vi "View Song Library Request by Album.vi"(8 "error in (no error)":errorcluster, 9 "Artist":string, 10 "Album":string, 11 "MusicManagerActor in":refnum<class "MusicManagerActor.lvclass">) -> (0 "error out":errorcluster, 3 "MusicManagerActor out":refnum<class "MusicManagerActor.lvclass">)   [LabVIEW 2015, in "MusicManagerActor.lvlib" / "MusicManagerActor.lvclass"]
uses:
  MusicManagerActor.lvclass
  MusicManagerActor.lvclass/MusicManagerActor.ctl
  file/MusicElement/Album/Album.lvclass/Album.ctl
  file/MusicElement/MusicElementLibrary/SongLibrary/SongLibrary.lvclass
  SongBrowserActor/SongBrowserActor Messages/Display Song Library Msg/Display Song Library Msg.lvclass
  file/MusicElement/MusicElementLibrary/MusicLibrary/MusicLibrary.lvclass
  SongQueueActor/SongQueueActor Messages/Set Visibility Of Queue List Msg/Set Visibility Of Queue List Msg.lvclass
  file/MusicElement/Album/Album.lvclass
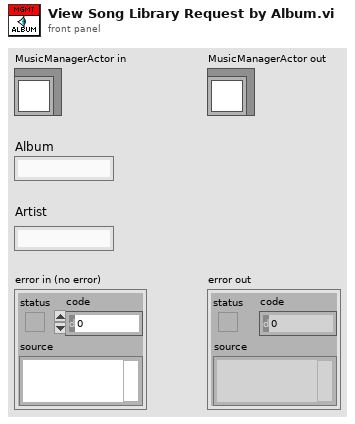
[diagram p1: front panel]
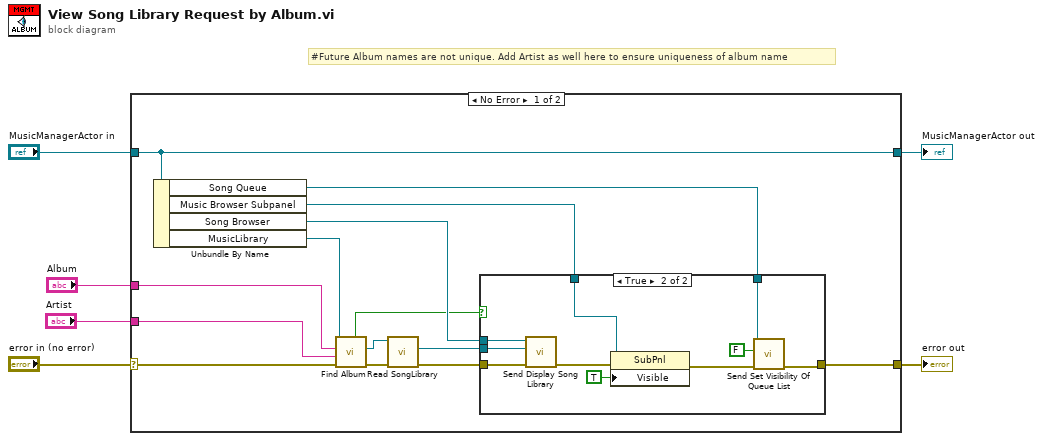
[diagram p0: block diagram]
diagram:
  # "#Future Album names are not unique. Add Artist as well here to ensure uniqueness of album name"
  n1 = case shown="No Error" "error in (no error)" {
    selector: "error in (no error)" -> [w16 w33]
    tunnel: [w19 w33] -> w5
    tunnel: [w20 w32] -> w3
    tunnel: "MusicManagerActor in" -> [w20 w32]
    tunnel: "Album" -> [w14 _]
    tunnel: "Artist" -> [w7 _]
    frame No Error {
      n2 = Unbundle By Name(w20) -> ("Song Queue"=w12:refnum<class "Message Enqueuer.lvclass">, "Music Browser Subpanel"=w18:refnum<vi>, "Song Browser"=w17:refnum<class "Message Enqueuer.lvclass">, "MusicLibrary"=w15:refnum<class "MusicLibrary.lvclass">)
      n3 = call "Find Album.vi"("error in (no error)"=w16, "Artist"=w7, "Album"=w14, "MusicLibrary in"=w15) -> ("error out"=w11:errorcluster, "Album"=w10:refnum<class "Album.lvclass">, "Found?"=w13:bool)  [unwired: 4 in, 1 out]
      n4 = call "Read SongLibrary.vi"("error in (no error)"=w11, "Album in"=w10) -> ("error out"=w8:errorcluster, "SongLibrary.lvclass"=w9:refnum<class "SongLibrary.lvclass">)  [unwired: 7 in, 1 out]
      n5 = case shown="True" w13 {
        tunnel: [w21 w24] -> w19
        tunnel: w18 -> [_ w31]
        tunnel: w17 -> [_ w28]
        tunnel: w9 -> [_ w27]
        tunnel: w8 -> [w21 w26]
        tunnel: w12 -> [_ w22]
        frame False {
        }
        frame True {
          n6 = call "Send Display Song Library.vi"("error in (no error)"=w26, "Song Library"=w27, "Message Enqueuer in"=w28) -> ("error out"=w29:errorcluster)  [unwired: 7 in, 1 out]
          n7 = property class="SubPnl"(reference=w31, error in=w29, "Visible"=TRUE) -> (error out=w23:errorcluster)  [unwired: 1 out]
          n8 = call "Send Set Visibility Of Queue List.vi"("error in (no error)"=w23, "Visible"=FALSE, "Message Enqueuer in"=w22) -> ("error out"=w24:errorcluster)  [unwired: 7 in, 1 out]
        }
      }
    }
    frame Error {
    }
  }
  "error out" <- w5
  "MusicManagerActor out" <- w3
